vi "Battery_Monitoring_Interface.vi"() -> ()   [LabVIEW 2026]
uses:
  <vilib>/numeric/Random Number (Range) U64.vi
  <vilib>/numeric/sub_Random U32.vi
panel:
  out "SoC (%)":dbl
  in  "?":bool
  out "Status":string
  out "Fault":bool
  out "Ok":bool
  out "Current Waveform Chart":dbl(graph)
  out "Voltage Waveform Chart":dbl(graph)
  out "Temperature Waveform Chart":dbl(graph)
  out "SoC":dbl(knob) scale=40.0..100.0
  out "Energy (Wh)":dbl
  out "Power (W)":dbl
  out "Temperature (*C)":dbl
  out "Current (A)":dbl
  out "Voltage (V)":dbl
  # "Battery Monitoring Interface"
  # "Battery Status"
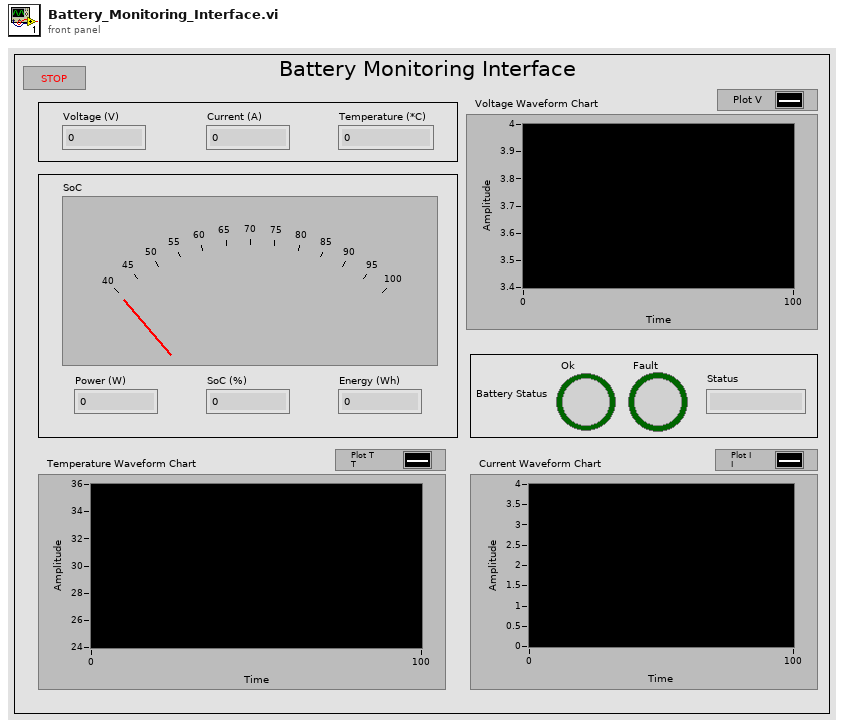
[diagram p1: front panel]
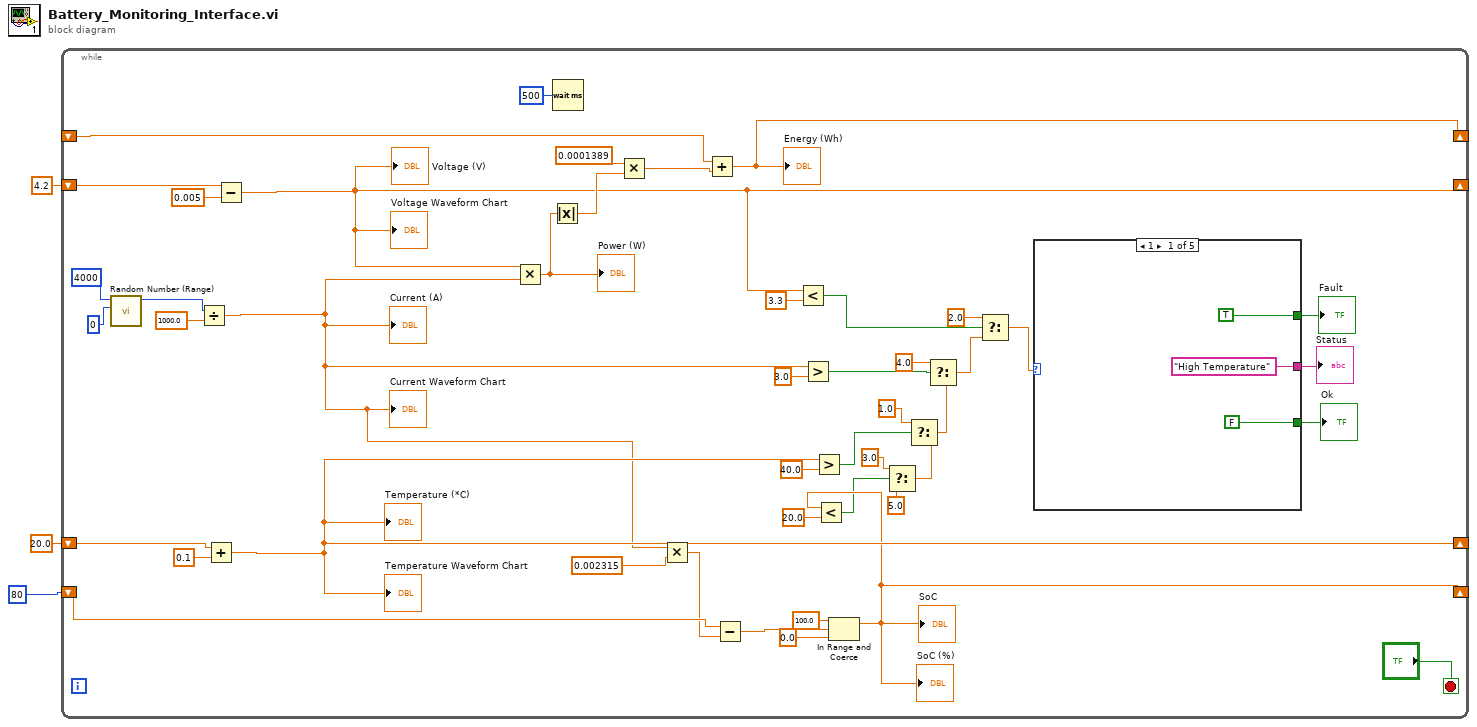
[diagram p0: block diagram]
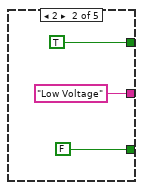
[diagram p2: hidden frame]
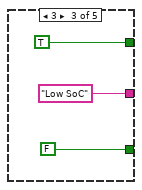
[diagram p3: hidden frame]
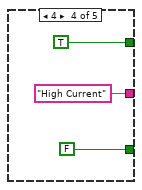
[diagram p4: hidden frame]
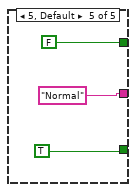
[diagram p5: hidden frame]
diagram:
  n1 = while {
    shift-right: [w45] -> _
    shift-left: _ -> [w46]
    shift-right: [w25] -> _
    shift-left: 80 -> [w43]
    shift-right: [w23] -> _
    shift-left: 4.2 -> [w35]
    shift-right: [w27] -> _
    shift-left: 20.0 -> [w33]
    stop <- "?" stop-if-true
    n2 = call-poly <vilib>:"Random Number (Range).vi"("lower bound (0)"=u64 0, "upper bound (100)"=u64 4000) -> ("number"=w30:u64)  [unwired: 9 in]
    n3 = Divide(x=w30, y=1000.0) -> (x/y=w21:dbl)
    "Current (A)" <- w21
    "Current Waveform Chart" <- w21
    n4 = Add(x=w33, y=0.1) -> (x+y=w27:dbl)
    "Temperature (*C)" <- w27
    "Temperature Waveform Chart" <- w27
    n5 = Subtract(x=w35, y=0.005) -> (x-y=w23:dbl)
    "Voltage (V)" <- w23
    "Voltage Waveform Chart" <- w23
    n6 = Multiply(x=w23, y=w21) -> (x*y=w40:dbl)
    "Power (W)" <- w40
    n7 = Absolute Value(x=w40) -> (abs(x)=w41:dbl)
    n8 = Wait (ms)(milliseconds to wait=u32 500) -> ()  [unwired: 1 out]
    n9 = Multiply(x=0.0001389, y=w41) -> (x*y=w47:dbl)
    n10 = Multiply(x=w21, y=0.002315) -> (x*y=w42:dbl)
    n11 = Add(x=w46, y=w47) -> (x+y=w45:dbl)
    "Energy (Wh)" <- w45
    n12 = Subtract(x=w43, y=w42) -> (x-y=w37:dbl)
    n13 = Less?(x=w23, y=3.3) -> (x < y?=w19:bool)
    n14 = Greater?(x=w21, y=3.0) -> (0:w17:bool)
    n15 = Greater?(x=w27, y=40.0) -> (0:w14:bool)
    n16 = In Range and Coerce(upper limit=100.0, x=w37, lower limit=0.0) -> (coerced(x)=w25:dbl)  [unwired: 1 out]
    "SoC" <- w25
    "SoC (%)" <- w25
    n17 = Less?(x=w25, y=20.0) -> (x < y?=w12:bool)
    n18 = Select(t=3.0, s=w12, f=5.0) -> (s? t:f=w10:dbl)
    n19 = Select(t=1.0, s=w14, f=w10) -> (s? t:f=w8:dbl)
    n20 = Select(t=4.0, s=w17, f=w8) -> (s? t:f=w16:dbl)
    n21 = Select(t=2.0, s=w19, f=w16) -> (s? t:f=w5:dbl)
    n22 = case shown="1" w5 {
      tunnel: [TRUE ("Fault") TRUE ("Fault") TRUE ("Fault") TRUE ("Fault") FALSE ("Fault")] -> w7
      tunnel: [FALSE ("Ok") FALSE ("Ok") FALSE ("Ok") FALSE ("Ok") TRUE ("Ok")] -> w6
      tunnel: ["High Temperature" ("Status") "Low Voltage" ("Status") "Low SoC" ("Status") "High Current" ("Status") "Normal" ("Status")] -> w4
      frame 1 {
      }
      frame 2 {
      }
      frame 3 {
      }
      frame 4 {
      }
      frame 5, Default {
      }
    }
    "Status" <- w4
    "Ok" <- w6
    "Fault" <- w7
  }
